vi "Write Map.vi"(8 "error in (no error)":errorcluster, 10 "Map":u16[][](array[numeric]), 11 "TrafficMap in":refnum<class "TrafficMap.lvclass">) -> (0 "error out":errorcluster, 3 "TrafficMap out":refnum<class "TrafficMap.lvclass">)   [LabVIEW 2017, in "TrafficMap.lvclass"]
uses:
  TrafficMap.lvclass
  TrafficMap.lvclass/TrafficMap.ctl
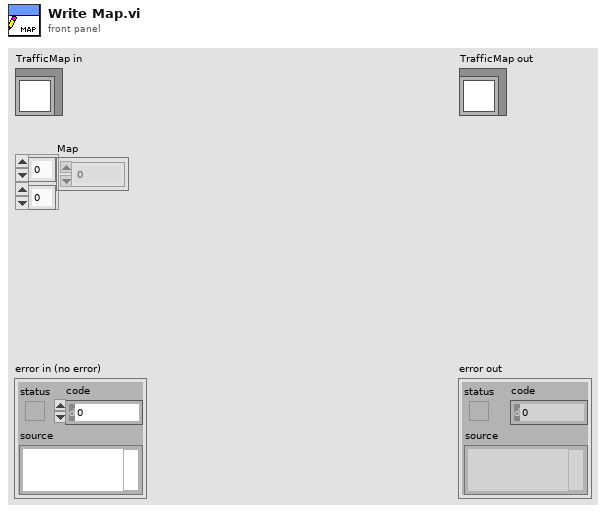
[diagram p1: front panel]
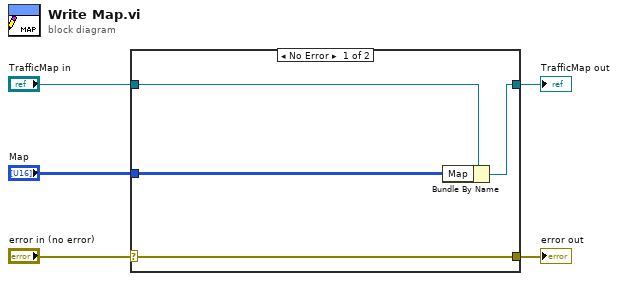
[diagram p0: block diagram]
diagram:
  n1 = case shown="No Error" "error in (no error)" {
    selector: "error in (no error)" -> [w9 w10]
    tunnel: [w9 w10] -> w4
    tunnel: [w7 w11] -> w2
    tunnel: "TrafficMap in" -> [w8 w11]
    tunnel: "Map" -> [w6 _]
    frame No Error {
      n2 = Bundle By Name(cluster=w8, "Map"=w6) -> (w7:refnum<class "TrafficMap.lvclass">)
    }
    frame Error {
    }
  }
  "error out" <- w4
  "TrafficMap out" <- w2
